vi "Alternate Retardance.vi"(0 "LCD Retarder in":refnum<class "LCD Retarder.lvclass">, 5 "Retardance 1":dbl, 7 "Retardance 2":dbl, 9 "Frequency":dbl, 11 "error in (no error)":errorcluster, 12 "Cycles":i32) -> (4 "LCD Retarder out":refnum<class "LCD Retarder.lvclass">, 8 "Current Retardance":dbl[unit] format="%#_6e", 15 "error out":errorcluster)   [LabVIEW 2009, in "LCD Retarder.lvclass"]
uses:
  LCD Retarder.lvclass
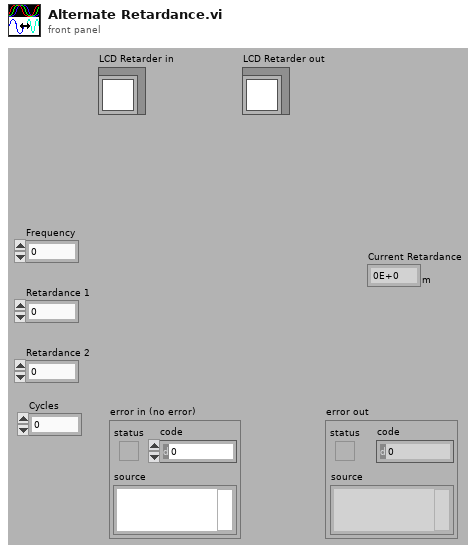
[diagram p1: front panel]
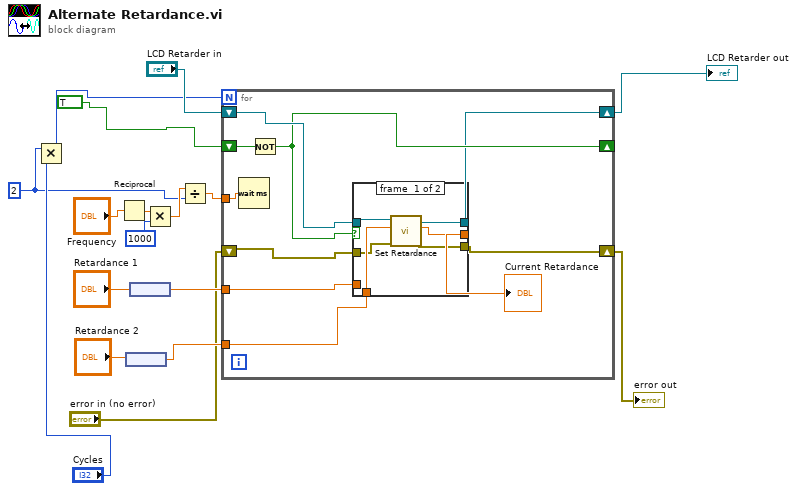
[diagram p0: block diagram]
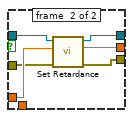
[diagram p2: hidden frame]
diagram:
  w1 = 2
  n1 = Multiply(x=w1, y="Cycles") -> (x*y=w4:i32)
  n2 = Reciprocal(x="Frequency") -> (1/x=w12:dbl)
  n3 = node("Retardance 2") -> (w10:dbl[unit])
  n4 = node("Retardance 1") -> (w15:dbl[unit])
  n5 = Multiply(x=w12, y=1000) -> (x*y=w2:dbl)
  n6 = Divide(x=w2, y=w1) -> (x/y=w3:dbl)
  n7 = for {
    N: w4 -> [_]
    tunnel: w15 -> [w26]
    tunnel: w3 -> [w24]
    tunnel: w10 -> [w23]
    shift-right: [w20] -> _
    shift-left: TRUE -> [w21]
    shift-right: [w25] -> w7
    shift-left: "error in (no error)" -> [w19]
    shift-right: [w18] -> w5
    shift-left: "LCD Retarder in" -> [w27]
    n8 = Wait (ms)(milliseconds to wait=w24) -> ()  [unwired: 1 out]
    n9 = Not(x=w21) -> (.not. x?=w20:bool)
    n10 = case shown="True" w20 {
      tunnel: w27 -> [w29 w35]
      tunnel: [w33 w39] -> w18
      tunnel: [w31 w37] -> w25
      tunnel: w26 -> [_ w36]
      tunnel: w23 -> [w30 _]
      tunnel: [w32 w38] -> w22
      tunnel: w19 -> [w28 w34]
      frame #0 {
        n11 = call "Set Retardance.vi"("errorIN"=w28, "Retardance"=w30, "LCD in"=w29) -> ("errorOUT"=w31:errorcluster, "Retardance out"=w32:dbl[unit], "LCD out"=w33:refnum<class "LCD Retarder.lvclass">)  [unwired: 6 in]
      }
      frame #1 {
        n12 = call "Set Retardance.vi"("errorIN"=w34, "Retardance"=w36, "LCD in"=w35) -> ("errorOUT"=w37:errorcluster, "Retardance out"=w38:dbl[unit], "LCD out"=w39:refnum<class "LCD Retarder.lvclass">)  [unwired: 6 in]
      }
    }
    "Current Retardance" <- w22
  }
  "error out" <- w7
  "LCD Retarder out" <- w5
